vi "Calibragem_bob.vi"() -> ()   [LabVIEW 2013]
uses:
  <vilib>/Analysis/baseanly.llb/Mean (DBL).vi
  <vilib>/Analysis/NI_AALBase.lvlib
  <vilib>/gmath/NI_Gmath.lvlib
panel:
  in  "Amostra":dbl=100.0
  out "Erro da média":dbl
  out "Desvio":dbl
  out "Média":dbl
  out "Dados brutos":dbl(graph)
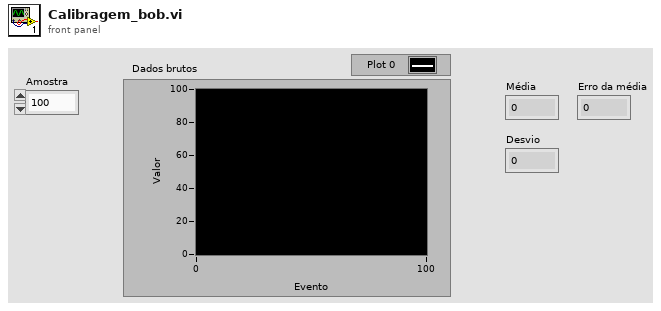
[diagram p1: front panel]
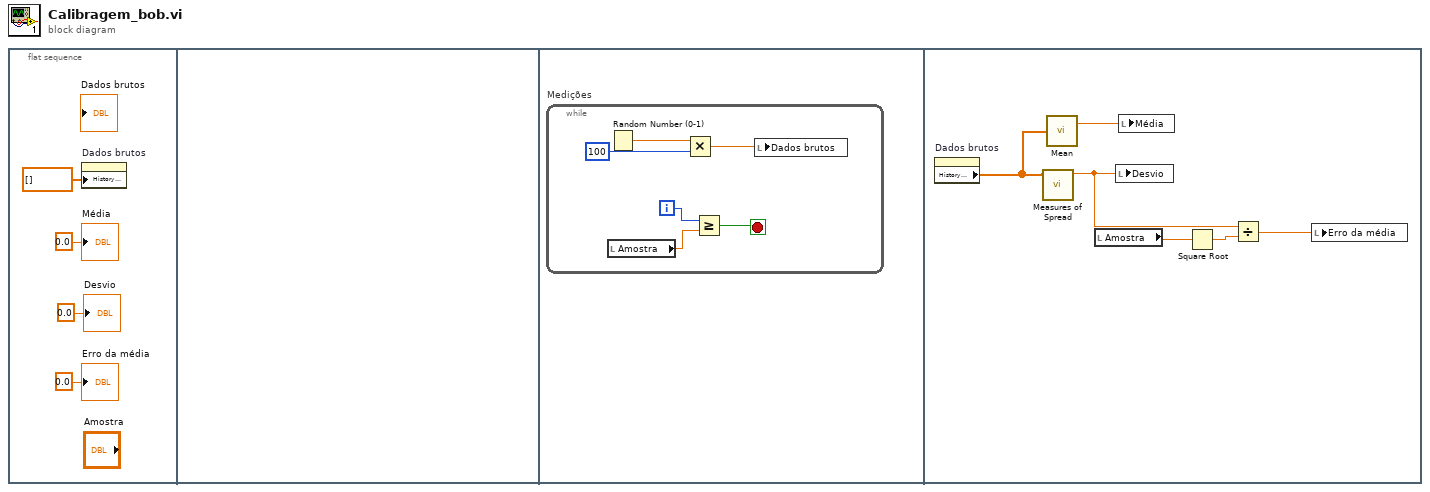
[diagram p0: block diagram]
diagram:
  n1 = flat-sequence {
    frame #0 {
      n2 = property on="Dados brutos" class="WFChart (strict)"("History Data"=dbl[] []) -> ()  [unwired: 2 in, 2 out]
      "Média" <- 0.0 ("Média")
      "Desvio" <- 0.0 ("Desvio")
      "Erro da média" <- 0.0 ("Erro da média")
    }
    frame #1 {
    }
    frame #2 {
      n3 = while "Medições" {
        i -> [w10]
        stop <- w9 stop-if-true
        n4 = Random Number (0-1)() -> (number: 0 to 1=w8:dbl)
        n5 = local read "Amostra"() -> (w5:dbl)
        n6 = Multiply(x=w8, y=100) -> (x*y=w6:dbl)
        n7 = Greater Or Equal?(x=w10, y=w5) -> (x >= y?=w9:bool)
        n8 = local write "Dados brutos"(w6) -> ()
      }
    }
    frame #3 {
      n9 = property on="Dados brutos" class="WFChart (strict)"() -> ("History Data"=w11:dbl[])  [unwired: 2 in, 2 out]
      n10 = call <vilib>:"Measures of Spread.vi"("x array"=w11) -> ("spread value"=w15:dbl)  [unwired: 9 in, 1 out]
      n11 = call-poly <vilib>:"Mean.vi"("X"=w11) -> ("mean"=w16:dbl)  [unwired: 1 out]
      n12 = local read "Amostra"() -> (w13:dbl)
      n13 = local write "Desvio"(w15) -> ()
      n14 = local write "Média"(w16) -> ()
      n15 = Square Root(x=w13) -> (sqrt(x)=w12:dbl)
      n16 = Divide(x=w15, y=w12) -> (x/y=w14:dbl)
      n17 = local write "Erro da média"(w14) -> ()
    }
  }
